vi "树控件拖动功能（内置数据源）.vi"() -> ()   [LabVIEW 2012, in "Tree Tools.lvlib"]
uses:
  Tree Tools.lvlib
  <vilib>/Analysis/NI_AALBase.lvlib
panel:
  out "波形图":dbl[](graph)
  out "波形数据":string[][](table)
  in  "停止":bool
  in  "选择波形拖动":string(tree)="猪八戒_1"
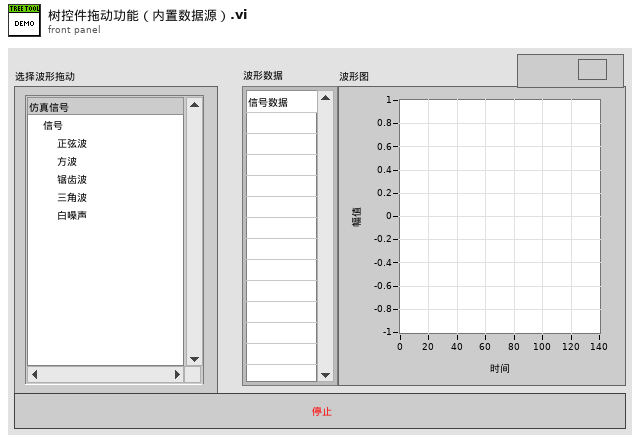
[diagram p1: front panel]
types:
  T1 = cluster{"data name":string, "drag data":variant}[]
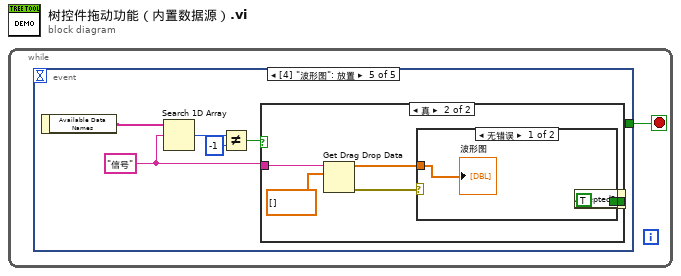
[diagram p0: block diagram]
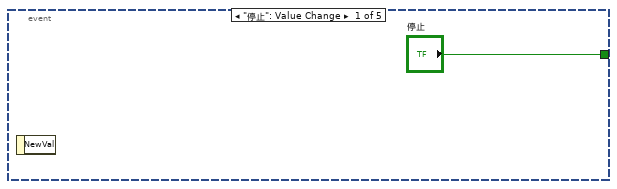
[diagram p2: hidden frame]
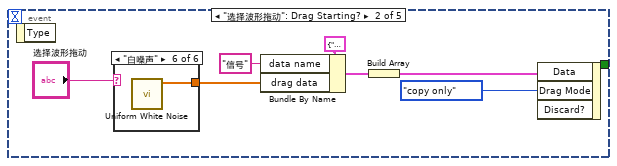
[diagram p3: hidden frame]
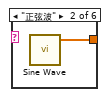
[diagram p5: hidden frame]
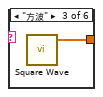
[diagram p6: hidden frame]
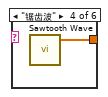
[diagram p7: hidden frame]
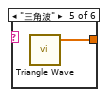
[diagram p8: hidden frame]
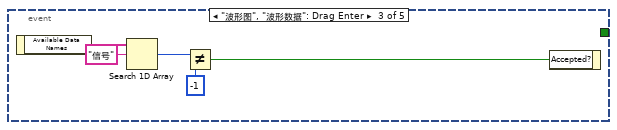
[diagram p9: hidden frame]
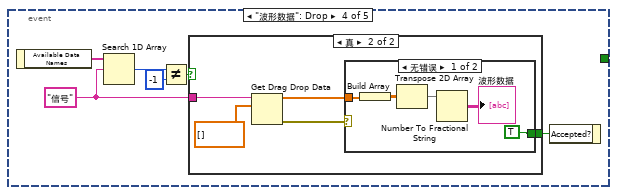
[diagram p10: hidden frame]
diagram:
  n1 = while {
    stop <- w1 stop-if-true
    n2 = event shown="[4] \"波形图\": 放置" {
      selector: _ -> [_ _ _ _ _]
      dyn-events: _ -> [_ _ _ _ _]
      timeout: _ -> [_ _ _ _ _]
      tunnel: ["停止" _ _ _ _] -> w1
      event "停止": Value Change {
        n3 = event-data() -> ()  [unwired: 1 in, 1 out]
      }
      event "选择波形拖动": Drag Starting? {
        n4 = event-data() -> ()  [unwired: 1 in, 1 out]
        n5 = case shown="\"白噪声\"" "选择波形拖动" {
          tunnel: [_ w10 w11 w12 w13 w14] -> w6
          frame "信号", Default {
          }
          frame "正弦波" {
            n6 = call <vilib>:"Sine Wave.vi"() -> ("sine wave"=w10:dbl[])  [unwired: 5 in, 2 out]
          }
          frame "方波" {
            n7 = call <vilib>:"Square Wave.vi"() -> ("square wave"=w11:dbl[])  [unwired: 6 in, 2 out]
          }
          frame "锯齿波" {
            n8 = call <vilib>:"Sawtooth Wave.vi"() -> ("sawtooth wave"=w12:dbl[])  [unwired: 5 in, 2 out]
          }
          frame "三角波" {
            n9 = call <vilib>:"Triangle Wave.vi"() -> ("triangle wave"=w13:dbl[])  [unwired: 5 in, 2 out]
          }
          frame "白噪声" {
            n10 = call <vilib>:"Uniform White Noise.vi"() -> ("uniform white noise"=w14:dbl[])  [unwired: 10 in, 1 out]
          }
        }
        n11 = Bundle By Name(cluster=cluster{"data name":string, "drag data":variant} {"data name"="", "drag data"=variant}, "data name"="信号", "drag data"=w6) -> (w5:cluster{"data name":string, "drag data":variant})
        n12 = Build Array(w5) -> (w4:T1)
        n13 = event-data("Data"=w4, "Drag Mode"=enum32{"copy or move", "copy only", "move only"}."copy only" ("拖曳模式")) -> ()  [unwired: 2 in, 1 out]
      }
      event "波形图", "波形数据": Drag Enter {
        n14 = event-data() -> ("Available Data Names"=w19:string[])  [unwired: 1 in]
        n15 = Search 1D Array(1D array=w19, element="信号" ("元素")) -> (index of element=w17:i32)  [unwired: 1 in]
        n16 = Not Equal?(x=w17, y=-1) -> (x != y?=w15:bool)
        n17 = event-data("Accepted?"=w15) -> ()  [unwired: 1 in, 1 out]
      }
      event "波形数据": Drop {
        w21 = "信号" ("element")
        n18 = event-data() -> ("Available Data Names"=w23:string[])  [unwired: 1 in]
        n19 = Search 1D Array(1D array=w23, element=w21) -> (index of element=w24:i32)  [unwired: 1 in]
        n20 = Not Equal?(x=w24, y=-1) -> (x != y?=w22:bool)
        n21 = case shown="真" w22 {
          tunnel: w21 -> [_ w30]
          tunnel: [_ w26] -> w20
          frame False {
          }
          frame True {
            n22 = Get Drag Drop Data(8:dbl[] [], 9:w30) -> (0:w28:errorcluster, 3:w27:dbl[])  [unwired: 1 in]
            n23 = case shown="无错误" w28 {
              tunnel: w27 -> [w35 _]
              tunnel: [TRUE _] -> w26
              frame No Error {
                n24 = Build Array(w35) -> (w32:dbl[][])
                n25 = Transpose 2D Array(2D array=w32) -> (transposed array=w31:dbl[][])
                n26 = Number To Fractional String(number=w31) -> (F-format string=→"波形数据":string[][])  [unwired: 3 in]
              }
              frame Error {
              }
            }
          }
        }
        n27 = event-data("Accepted?"=w20) -> ()  [unwired: 1 in, 1 out]
      }
      event "波形图": Drop {
        w36 = "信号" ("element")
        n28 = event-data() -> ("Available Data Names"=w38:string[])  [unwired: 1 in]
        n29 = Search 1D Array(1D array=w38, element=w36) -> (index of element=w39:i32)  [unwired: 1 in]
        n30 = Not Equal?(x=w39, y=-1) -> (x != y?=w37:bool)
        n31 = case shown="真" w37 {
          tunnel: w36 -> [_ w45]
          tunnel: [_ w41] -> _
          frame False {
          }
          frame True {
            n32 = Get Drag Drop Data(8:dbl[] [], 9:w45) -> (0:w43:errorcluster, 3:w42:dbl[])  [unwired: 1 in]
            n33 = case shown="无错误" w43 {
              tunnel: w42 -> [w46 _]
              tunnel: [TRUE _] -> w41
              frame No Error {
                "波形图" <- w46
              }
              frame Error {
              }
            }
          }
        }
        n34 = event-data() -> ()  [unwired: 2 in, 1 out]
      }
    }
  }
